vi "Set Numeric.vi"(8 "error in (no error)":errorcluster, 10 "Numeric":dbl, 11 "Element A in":refnum<class "Element B.lvclass">) -> (0 "error out":errorcluster, 3 "Element A out":refnum<class "Element B.lvclass">)   [LabVIEW 2014, in "Array Example.lvlib" / "Element B.lvclass"]
uses:
  Element B.lvclass
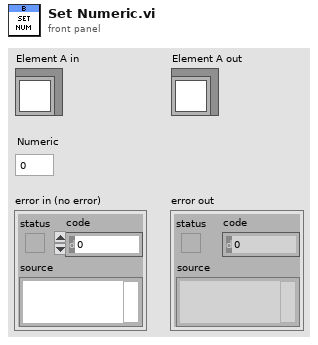
[diagram p1: front panel]
types:
  T1 = typedef "Element B.lvclass/Ref.ctl" = cluster{"Value":dbl}
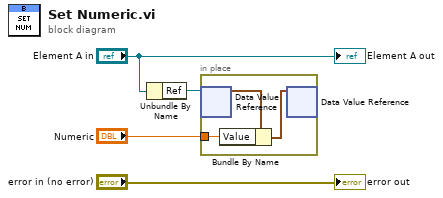
[diagram p0: block diagram]
diagram:
  n1 = Unbundle By Name("Element A in") -> ("Ref"=w3:refnum<data-value>)
  n2 = in-place {
    in-place-border: "Numeric" -> [w5]
    n3 = in-place-dvr #1(w3) -> (w7:T1)  [unwired: 1 out]
    n4 = Bundle By Name(cluster=w7, "Value"=w5) -> (w6:T1)
    n5 = in-place-dvr #1(w6) -> ()  [unwired: 2 out]
  }
  "error out" <- "error in (no error)"
  "Element A out" <- "Element A in"
